vi "niDTS BT INSTR TX Configure PortMapping.vi"(8 "error in (no error)":errorcluster, 11 "niDTS BT INSTR TX in":refnum<class "niDTS BT INSTR TX.lvclass">) -> (0 "error out":errorcluster, 3 "niDTS BT INSTR TX out":refnum<class "niDTS BT INSTR TX.lvclass">)   [LabVIEW 2015, in "niDTS BT.lvlib" / "niDTS BT INSTR TX.lvclass"]
uses:
  niDTS BT INSTR TX.lvclass
  niDTS BT INSTR TX.lvclass/niDTS BT INSTR TX.ctl
  RiviInstDriver/niRfsaBT/Objects/niRfsaBt.lvclass
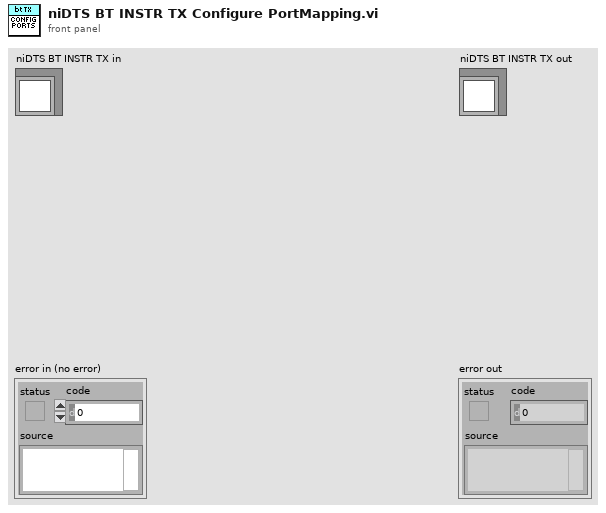
[diagram p1: front panel]
types:
  T1 = typedef "niRfsaBT.lvclass/niRfsaBT INC Handle.ctl" = refnum<data-value>
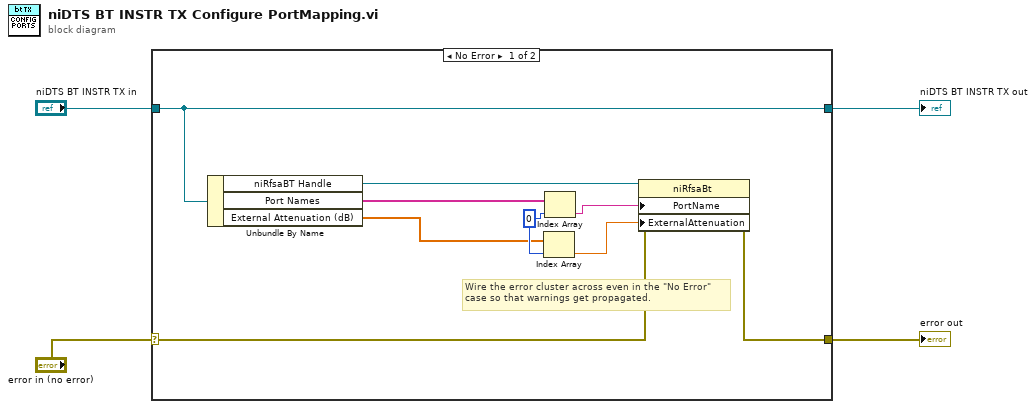
[diagram p0: block diagram]
diagram:
  n1 = case shown="No Error" "error in (no error)" {
    selector: "error in (no error)" -> [w12 w15]
    tunnel: [w11 w15] -> w3
    tunnel: [w13 w14] -> w1
    tunnel: "niDTS BT INSTR TX in" -> [w13 w14]
    frame No Error {
      w7 = 0 ("index")
      # "Wire the error cluster across even in the \"No Error\"\ncase so that warnings get propagated."
      n2 = Unbundle By Name(w13) -> ("niRfsaBT Handle"=w10:T1, "Port Names"=w9:string[], "External Attenuation (dB)"=w6:dbl[])
      n3 = Index Array(array=w6, index=w7) -> (element=w5:dbl)
      n4 = Index Array(array=w9, index=w7) -> (element=w8:string)
      n5 = property class="niRfsaBt"(reference=w10, error in=w12, "PortName"=w8, "ExternalAttenuation"=w5) -> (error out=w11:errorcluster)  [unwired: 1 out]
    }
    frame Error {
    }
  }
  "error out" <- w3
  "niDTS BT INSTR TX out" <- w1
